vi "libssh2_session_disconnect.vi"(8 "error in (no error)":errorcluster, 10 "description":string, 11 "session":u64) -> (0 "error out":errorcluster, 3 "return value":i32)   [LabVIEW 2013, in "libssh2.lvlib"]
uses:
  libssh2.lvlib
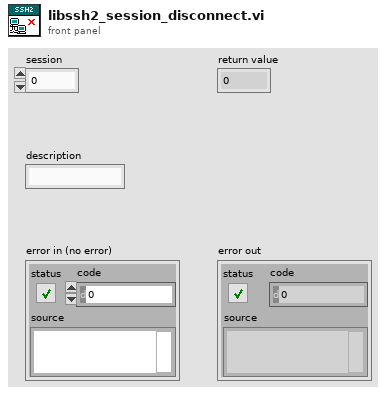
[diagram p1: front panel]
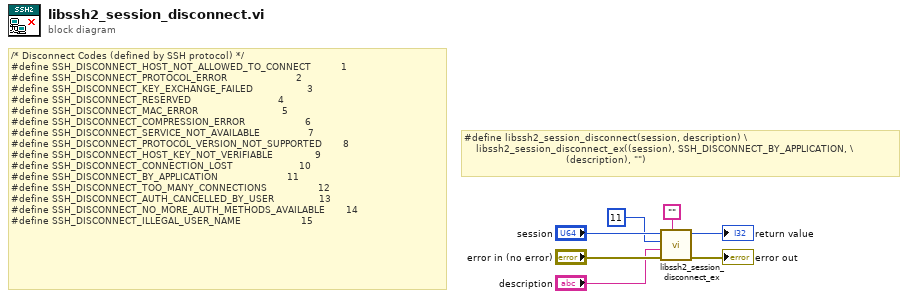
[diagram p0: block diagram]
diagram:
  # "/* Disconnect Codes (defined by SSH protocol) */\n#define SSH_DISCONNECT_HOST_NOT_ALLOWED_TO_CONNECT          1\n#define SSH_DISCONNECT_PROTOCOL_ERROR                       2\n#define SSH_DISCONNECT_KEY_EXCHANGE_FAILED                  3\n#define SSH_DISCONNECT_RESERVED                             4\n#define SSH_DISCONNECT_MAC_ERROR                            5\n#define SSH_DISCONNECT_COMPRESSION_ERROR                    6\n#define SSH_DISCONNECT_SERVICE_NOT_AVAILABLE                7\n#define SSH_DISCONNECT_PROTOCOL_VERSION_NOT_SUPPORTED       8\n#define SSH_DISCONNECT_HOST_KEY_NOT_VERIFIABLE              9\n#define SSH_DISCONNECT_CONNECTION_LOST                      10\n#define SSH_DISCONNECT_BY_APPLICATION                       11\n#define SSH_DISCONNECT_TOO_MANY_CONNECTIONS                 12\n#define SSH_DISCONNECT_AUTH_CANCELLED_BY_USER               13\n#define SSH_DISCONNECT_NO_MORE_AUTH_METHODS_AVAILABLE       14\n#define SSH_DISCONNECT_ILLEGAL_USER_NAME                    15"
  # "#define libssh2_session_disconnect(session, description) \\\n    libssh2_session_disconnect_ex((session), SSH_DISCONNECT_BY_APPLICATION, \\\n                                  (description), \"\")"
  n1 = call "libssh2_session_disconnect_ex.vi"("lang"="", "error in (no error)"="error in (no error)", "description"="description", "reason"=11, "session"="session") -> ("error out"=→"error out":errorcluster, "return value"=→"return value":i32)  [unwired: 5 in]
